vi "BASIC_SUBVI_GaussianWhiteNoise.vi"(1 "Rnd 2":dbl, 2 "Rnd 1":dbl) -> (0 "NormalizedGaussianWhiteNoise":dbl)   [LabVIEW 2020]
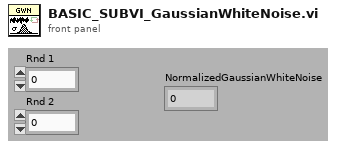
[diagram p1: front panel]
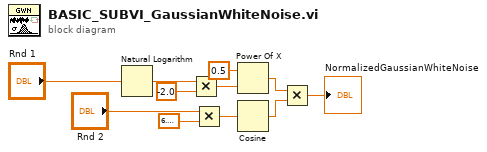
[diagram p0: block diagram]
diagram:
  n1 = Natural Logarithm(1:"Rnd 1") -> (0:w11:dbl)
  n2 = Multiply(x=w11, y=-2.0) -> (x*y=w9:dbl)
  n3 = Multiply(x="Rnd 2", y=6.283185307179586) -> (x*y=w6:dbl)
  n4 = Power Of X(1:w9, 2:0.5 ("y")) -> (0:w5:dbl)
  n5 = Cosine(x=w6) -> (cos(x)=w4:dbl)
  n6 = Multiply(x=w5, y=w4) -> (x*y=→"NormalizedGaussianWhiteNoise":dbl)
